vi "Create Config JSON.vi"() -> ()   [LabVIEW 2026]
uses:
  Plugin/AMS Power Supply Template/Configuration Params.ctl
  <vilib>/ADAS Replay HIL/Template Node/Plugin/Template Node/Common Configuration Params.ctl
  <vilib>/ADAS Replay HIL/AdasCommonUtilities/AdasCommonUtilities.lvlib
  8f15ed5a-ad49-4887-bb27-9da39d6e7646.vi
  C:/Program Files/National Instruments/AMS plugin/Capabilities/Capabilities/Utilities/Utilities.lvlib
  C:/Program Files/National Instruments/AMS plugin/Capabilities/Capabilities/High Level Capabilities/Power Supply Cluster/Power Supply Cluster.lvclass
  <vilib>/ADAS Replay HIL/Template Node/Plugin/Template Node/Template Node.lvclass
  Plugin/AMS Power Supply Template/AMS Power Supply Template.lvclass
panel:
  out "PAtools JSON":string
  in  "Create PAtools importable JSON?":bool=TRUE
  out "Version":string
  out "Generated JSON string":string
  out "error out":errorcluster
  in  "Custom Parameters":T1={"Common"={"Iteration Interval (s)"=0.001, "T0 (ns)"=0, "Priority"=100, "Processor"=-2, "Wait in Ready State"=TRUE}, "Amount of Channels"=1, "Address"=""} {"Common"."Iteration Interval (s)" format="%#_13g"}
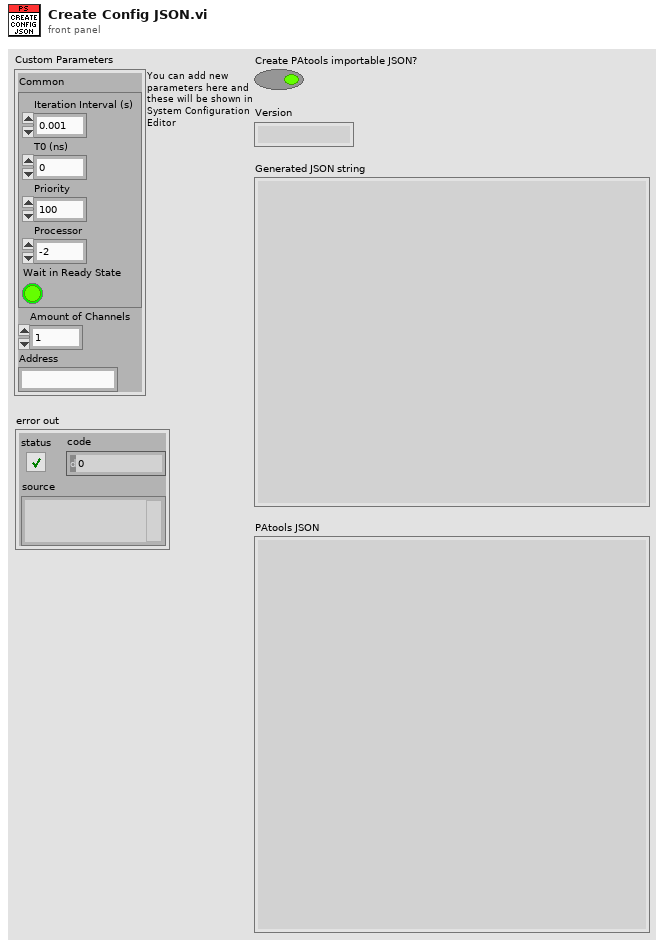
[diagram p1: front panel]
types:
  T1 = typedef "AMS Power Supply Template.lvlib/AMS Power Supply Template.lvclass/Configuration Params.ctl" = cluster{"Common":T2, "Amount of Channels":u32, "Address":string}
  T2 = typedef "Template Node.lvlib/Template Node.lvclass/Common Configuration Params.ctl" = cluster{"Iteration Interval (s)":dbl, "T0 (ns)":u64, "Priority":i32, "Processor":i32, "Wait in Ready State":bool}
  T3 = typedef "NI_App_Builder_API.lvlib/Build Specification Version.ctl" = cluster{"Major":u16, "Minor":u16, "Fix":u16, "Build":u16}
  T4 = typedef "Utilities.lvlib/Channel.ctl" = cluster{"Title":string, "SubTitle":string[], "Consumer?":bool, "Name":string, "Description":string, "Size":i32, "OffSets":i32[], "DataType":string[], "DefaultValue":dbl[]}
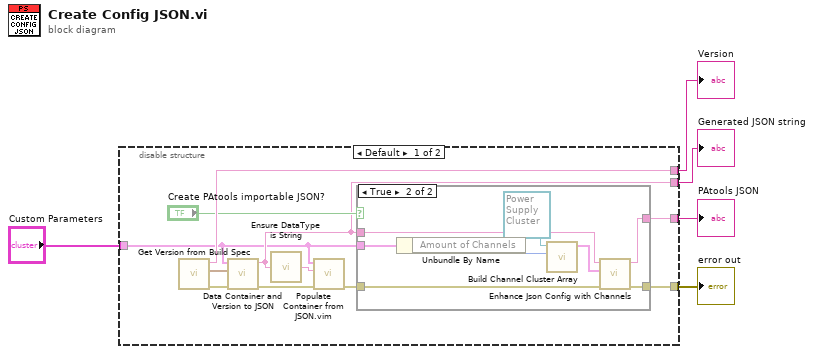
[diagram p0: block diagram]
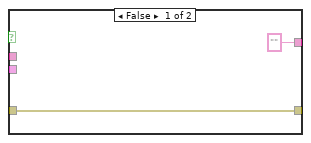
[diagram p2: hidden frame]
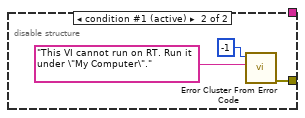
[diagram p3: hidden frame]
diagram:
  n1 = disable-structure shown="Default" {
    disable-tunnel: [w10 _] -> w5
    disable-tunnel: "Custom Parameters" -> [w6 _]
    disable-tunnel: [w8 w29] -> w3
    disable-tunnel: [w12 _] -> w2
    disable-tunnel: [w7 _] -> w1
    frame condition #0 {
      n2 = call "Get Version from Build Spec.vi"() -> ("error out"=w14:errorcluster, "Version"=w13:T3, "Version String"=w12:string)  [unwired: 8 in, 1 out]
      n3 = call <vilib>:"Data Container and Version to JSON.vi"("error in (no error)"=w14, "Version"=w13, "Container Variant"=w6) -> ("error out"=w16:errorcluster, "JSON string"=w10:string)  [unwired: 7 in]
      n4 = call <vilib>:"Ensure DataType is String.vi"("JSON In"=w10) -> ("JSON out"=w15:string)
      n5 = call "Populate Container from JSON.vim"("error in (no error)"=w16, "JSON string In"=w15, "Container In"=w6) -> ("error out"=w9:errorcluster)  [unwired: 6 in, 2 out]
      n6 = case shown="True" "Create PAtools importable JSON?" {
        tunnel: w10 -> [_ w26]
        tunnel: w9 -> [w18 w25]
        tunnel: [w18 w24] -> w8
        tunnel: ["" ("PAtools JSON") w23] -> w7
        tunnel: w6 -> [_ w22]
        frame False {
        }
        frame True {
          n7 = Unbundle By Name(w22) -> ("Amount of Channels"=w21:u32)
          n8 = call-dynamic "Build Channel Cluster Array.vi"("Power Supply Cluster.lvclass in"=refnum<class "Power Supply Cluster.lvclass"> refnum, "Channels Amount"=w21) -> ("Channels out"=w20:cluster{"Channels":T4[]})  [unwired: 8 in]
          n9 = call "Enhance Json Config with Channels.vi"("error in"=w25, "Channels"=w20, "Json Config"=w26) -> ("error out"=w24:errorcluster, "PAtools JSON"=w23:string)  [unwired: 7 in]
        }
      }
    }
    frame condition #1 (active) {
      n10 = call <vilib>:"Error Cluster From Error Code.vi"("error message (\"\")"="This VI cannot run on RT. Run it under \"My Computer\"." ("error message (\"\")"), "error code (0)"=-1) -> ("error out"=w29:errorcluster)  [unwired: 7 in]
    }
  }
  "Generated JSON string" <- w5
  "error out" <- w3
  "Version" <- w2
  "PAtools JSON" <- w1
